vi "tdmsViewer.vi"   [LabVIEW 2024]
uses:
  <vilib>/Utility/TDMS File Viewer/NI_TDMS File Viewer.lvlib
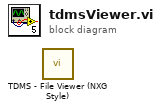
[diagram p0: block diagram]
diagram:
  n1 = call <vilib>:"TDMS - File Viewer (NXG Style).vi"() -> ()  [unwired: 10 in, 2 out]
